vi "cmd_start_server.vi"(8 "error in (no error)":errorcluster, 11 "JSON":string) -> (0 "error out":errorcluster)   [LabVIEW 2021]
doc: "Start server\n\n :param port: Specifies the port number"
uses:
  core/host_global_vars.vi
panel:
  in  "args":cluster{"port":u16}
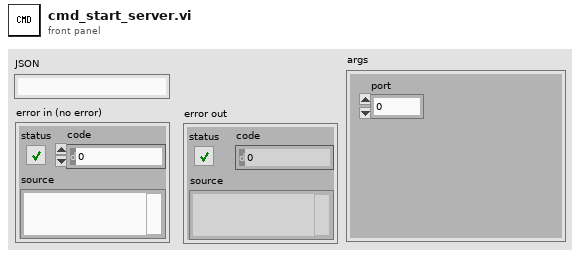
[diagram p1: front panel]
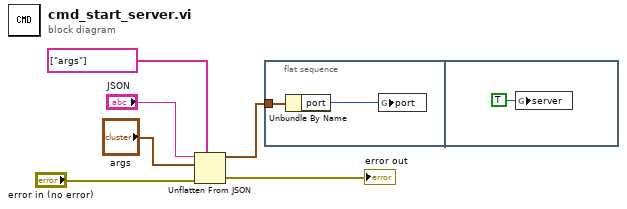
[diagram p0: block diagram]
diagram:
  n1 = Unflatten From JSON(path=string[] ["args"], JSON string="JSON", type and defaults="args", error in (no error)="error in (no error)") -> (value=w1:cluster{"port":u16}, error out=→"error out":errorcluster)  [unwired: 3 in]
  n2 = flat-sequence {
    tunnel: w1 -> [w8]
    frame #0 {
      n3 = Unbundle By Name(w8) -> ("port"=w7:u16)
      n4 = global write "host_global_vars.vi" "port"(w7) -> ()
    }
    frame #1 {
      n5 = global write "host_global_vars.vi" "server"(TRUE ("server")) -> ()
    }
  }
